vi "Demodulacja_DSBFC.vi"(6 "Parametry_sygnalu_nosnego":T1, 9 "Pasmo_przenoszenia":cluster{"f_L":dbl, "f_H":dbl}, 10 "Czestotliwosc_probkowania":dbl, 11 "Sygnal_zmodulowany":dbl[](array[numeric])) -> (3 "Sygnal_zdemodulowany":dbl[](array[numeric]))   [LabVIEW 2020]
doc: "VI demoduluje sygnal zmodulowany metoda DSBFC"
uses:
  Kontrolki/Parametry_cosinusa.ctl
  <vilib>/Analysis/3filter.llb/Filter Passband Type.ctl
  <vilib>/Analysis/3filter.llb/Butterworth Filter (DBL).vi
  <vilib>/Analysis/NI_AALBase.lvlib
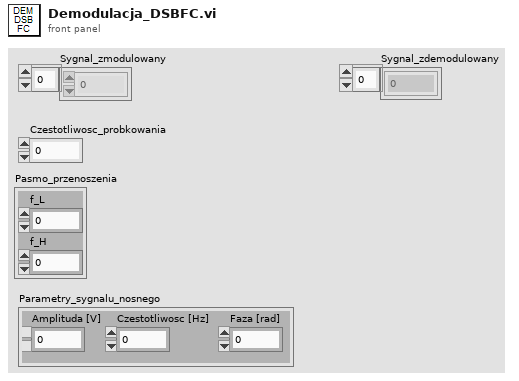
[diagram p1: front panel]
types:
  T1 = typedef "Parametry_cosinusa.ctl" = cluster{"Amplituda [V]":dbl, "Czestotliwosc [Hz] ":dbl, "Faza [rad]":dbl}
  T2 = typedef "NI_AALBase.lvlib/Filter Passband Type.ctl" = enum32{"Lowpass", "Highpass", "Bandpass", "Bandstop"}
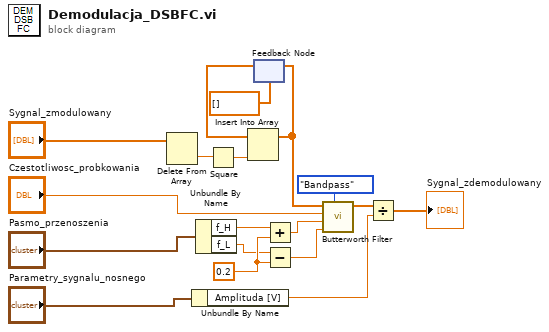
[diagram p0: block diagram]
diagram:
  w13 = 0.2
  n1 = Delete From Array(array="Sygnal_zmodulowany") -> (deleted portion=w7:dbl)  [unwired: 2 in, 1 out]
  n2 = Unbundle By Name("Parametry_sygnalu_nosnego") -> ("Amplituda [V]"=w1:dbl)
  n3 = Unbundle By Name("Pasmo_przenoszenia") -> ("f_H"=w10:dbl, "f_L"=w12:dbl)
  n4 = Square(x=w7) -> (x^2=w8:dbl)
  n5 = feedback #1(dbl[] []) -> (w18:dbl[])
  n6 = Insert Into Array(array=w18, new element=w8) -> (w17:dbl[])  [unwired: 1 in]
  n7 = feedback-in #1(w17) -> ()
  n8 = Add(x=w10, y=w13) -> (x+y=w11:dbl)
  n9 = Subtract(x=w12, y=w13) -> (x-y=w14:dbl)
  n10 = call-poly <vilib>:"Butterworth Filter.vi"("filter type"=Filter_Passband_Type."Bandpass", "low cutoff freq: fl"=w14, "high cutoff freq: fh"=w11, "sampling freq: fs"="Czestotliwosc_probkowania", "X"=w17) -> ("Filtered X"=w15:dbl[])  [unwired: 3 in, 1 out]
  n11 = Divide(x=w15, y=w1) -> (x/y=→"Sygnal_zdemodulowany":dbl[])
